vi "Write measurement type.vi"(8 "error in (no error)":errorcluster, 10 "measurement type":string, 11 "_dataProcessing in":refnum<class "_dataProcessing.lvclass">) -> (0 "error out":errorcluster, 3 "_dataProcessing out":refnum<class "_dataProcessing.lvclass">)   [LabVIEW 2019, in "_dataProcessing.lvlib" / "_dataProcessing.lvclass"]
uses:
  _dataProcessing.lvclass
  _dataProcessing.lvclass/_dataProcessing.ctl
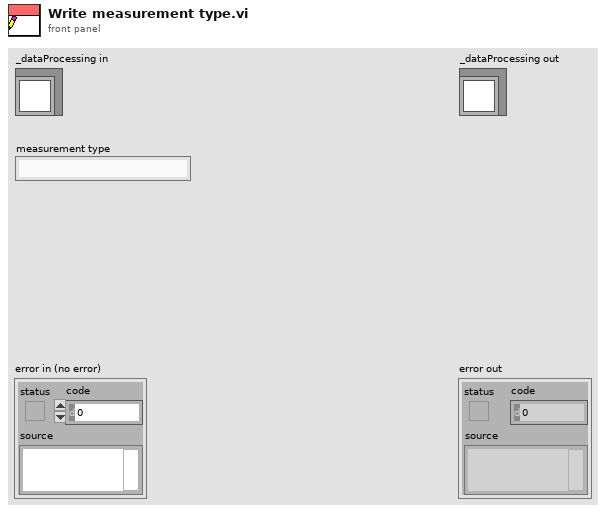
[diagram p1: front panel]
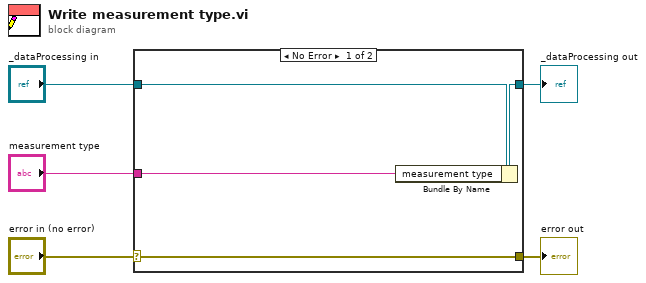
[diagram p0: block diagram]
diagram:
  n1 = case shown="No Error" "error in (no error)" {
    selector: "error in (no error)" -> [w9 w10]
    tunnel: [w9 w10] -> w4
    tunnel: [w7 w11] -> w2
    tunnel: "_dataProcessing in" -> [w8 w11]
    tunnel: "measurement type" -> [w6 _]
    frame No Error {
      n2 = Bundle By Name(cluster=w8, "measurement type"=w6) -> (w7:refnum<class "_dataProcessing.lvclass">)
    }
    frame Error {
    }
  }
  "error out" <- w4
  "_dataProcessing out" <- w2
